vi "Add (Elementwise) - C,CM.vi"(1 "Complex Matrix A":T1, 2 "Complex Scalar c":cdb) -> (0 "c + A":T1)   [LabVIEW 2017, in "NI_Matrix.lvlib"]
doc: "Computes the sum of the inputs."
uses:
  NI_Matrix.lvlib
  ComplexMatrix.ctl
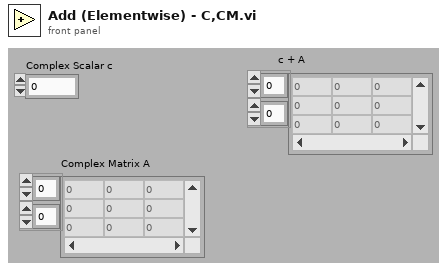
[diagram p1: front panel]
types:
  T1 = typedef "NI_Matrix.lvlib/ComplexMatrix.ctl" = cdb[][]
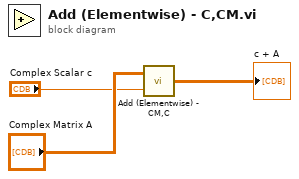
[diagram p0: block diagram]
diagram:
  n1 = call "Add (Elementwise) - CM,C.vi"("Complex Scalar c"="Complex Scalar c", "Complex Matrix A"="Complex Matrix A") -> ("A + c"=→"c + A":T1)
